vi "Heat Up Macro Prepare Data for Step.vi"(8 "Error In":errorcluster, 10 "Columns Too Search For":string[](array[string])=["System Time", "Draw Elapsed Time (s)", "Elapsed Time (s)", "UE - state (1/0 on off)", "LE - state (1/0 on off)", "Comp - state (1/0 on off)", "Fan  - state (1/0 on off)", "GALLONS", "FLOW(GPM)", "Intellifaucet Valve % Open", "Program Status", "Flow Events (Bit Encoded)"], 11 "HeatUp Raw Data Input":string[][](array[string])) -> (0 "Error Out":errorcluster, 2 "Heat Up Data with Only Selected Columns":string[][](array[string]))   [LabVIEW 2019]
uses:
  <vilib>/Utility/error.llb/DialogType.ctl
panel:
  out "index of element":i32
  out "In-Coming Headers":string[](array[string])
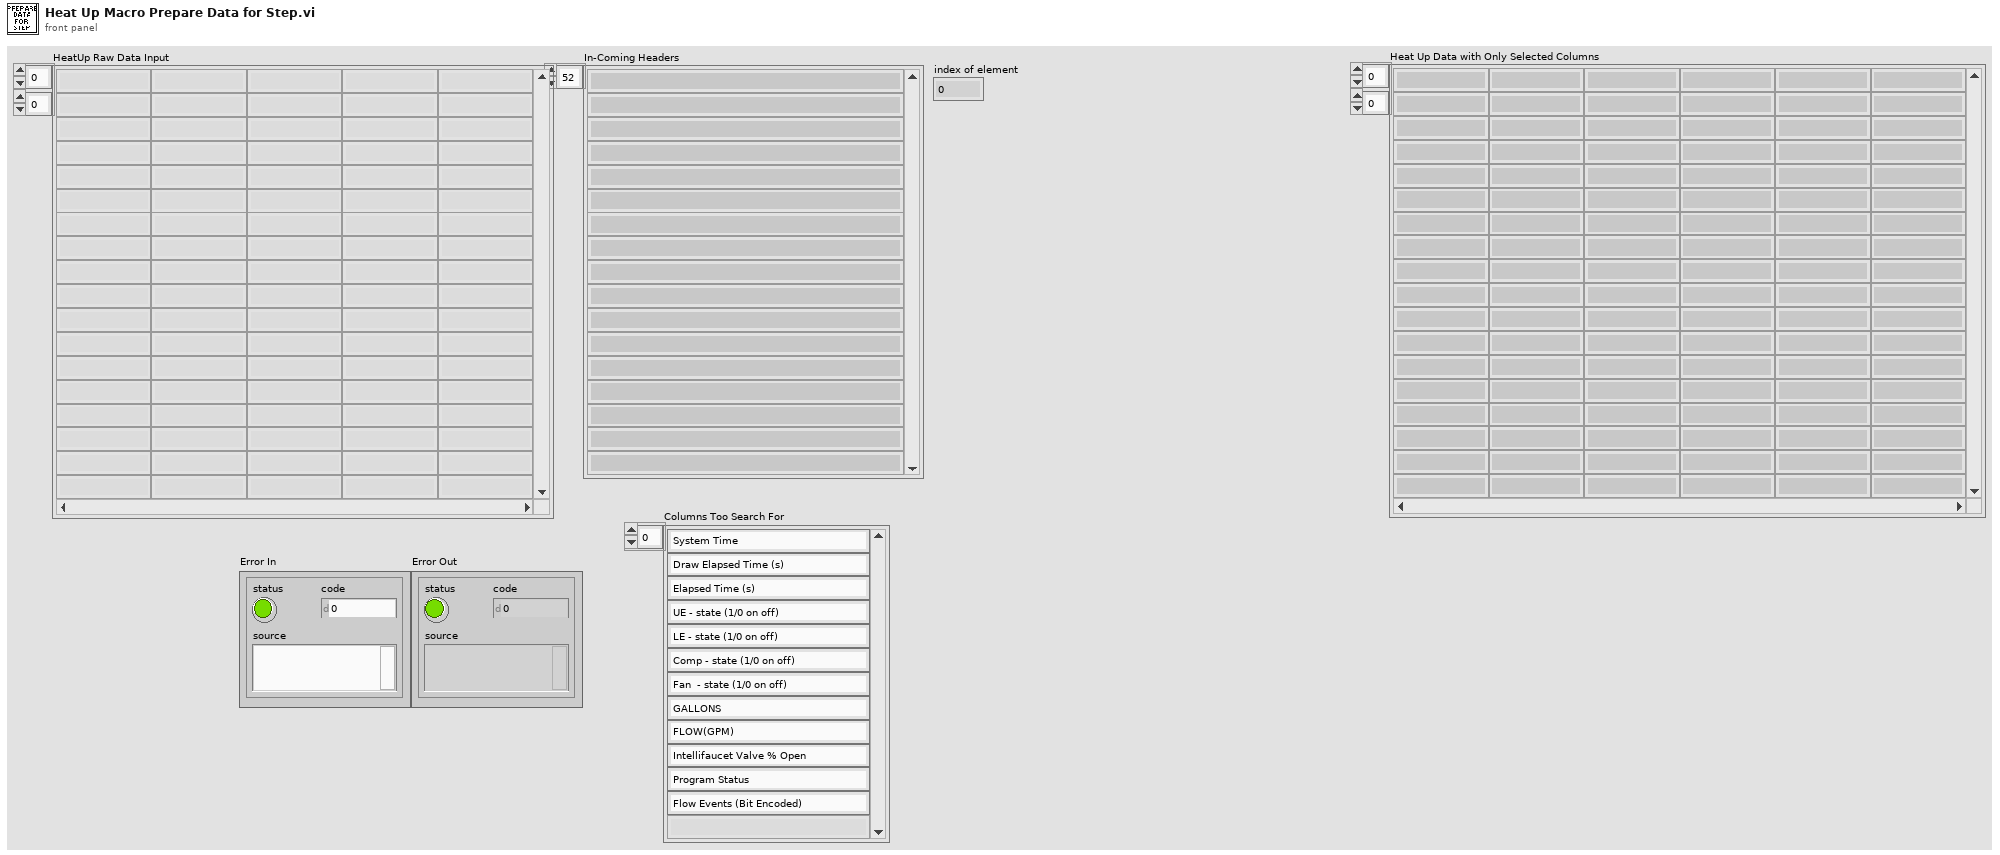
[diagram p1: front panel]
types:
  T1 = typedef "DialogType.ctl" = u16
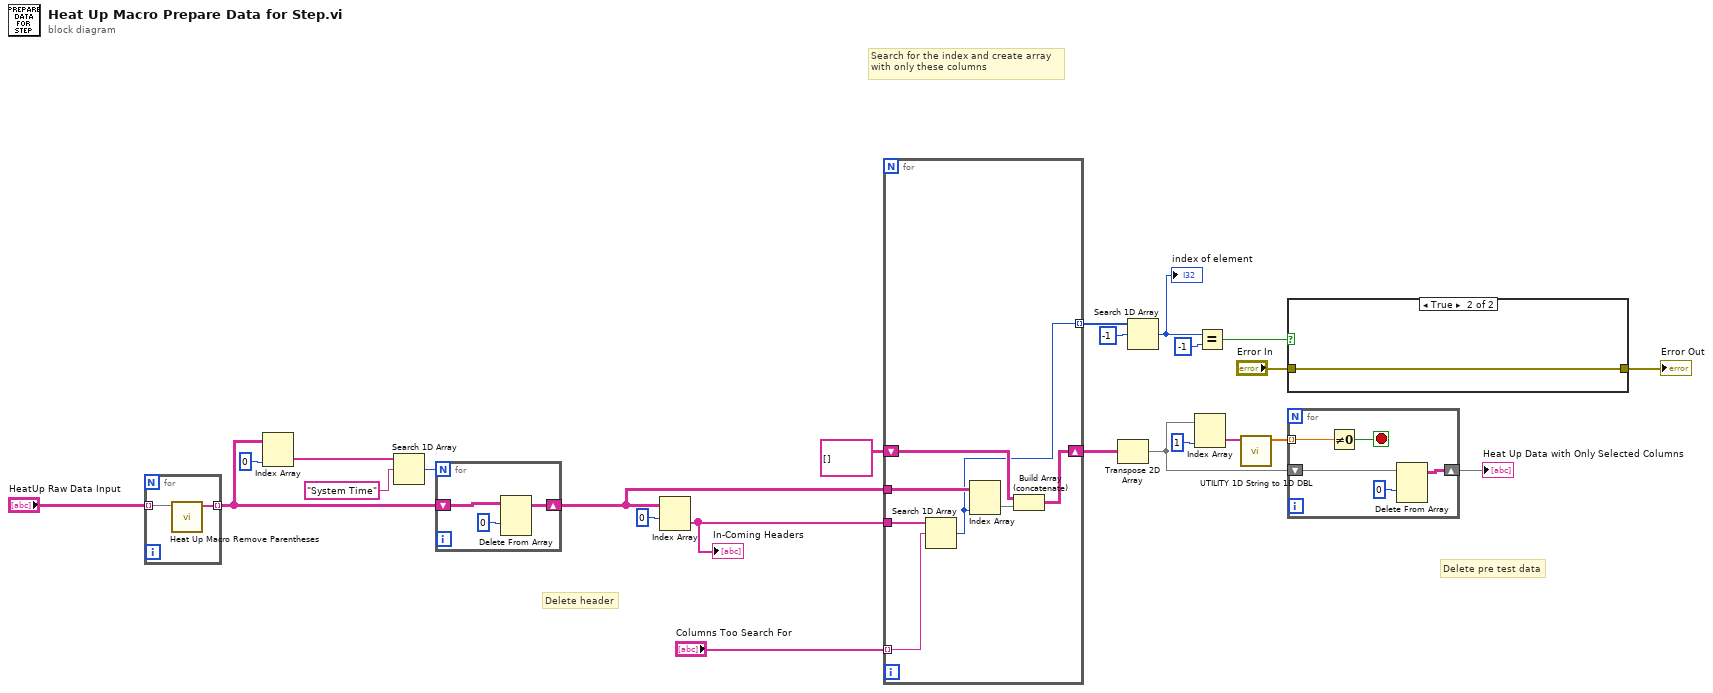
[diagram p0: block diagram]
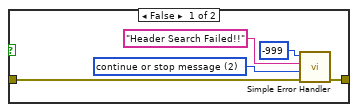
[diagram p2: hidden frame]
diagram:
  # "Delete pre test data"
  # "Delete header"
  # "Search for the index and create array\nwith only these columns"
  n1 = for {
    tunnel: "HeatUp Raw Data Input" -> [w26] mode=indexing
    tunnel: [w25] -> w1 mode=indexing
    n2 = call "Heat Up Macro Remove Parentheses.vi"("Input Array"=w26) -> ("Clean Array"=w25:string[])  [unwired: 10 in]
  }
  n3 = Index Array(array=w1, index (col)=0 ("disabled index (col)")) -> (element=w14:string[])  [unwired: 1 in]
  n4 = Search 1D Array(1D array=w14, element="System Time") -> (index of element=w12:i32)  [unwired: 1 in]
  n5 = for {
    N: w12 -> [_]
    shift-right: [w28] -> w18
    shift-left: w1 -> [w29]
    n6 = Delete From Array(array=w29, index (row)=0) -> (array with subset deleted=w28:string[][])  [unwired: 2 in, 1 out]
  }
  n7 = Index Array(array=w18, index (row)=0) -> (element=w3:string[])  [unwired: 1 in]
  "In-Coming Headers" <- w3
  n8 = for {
    tunnel: w3 -> [w31]
    shift-right: [w35] -> w21
    shift-left: string[][] [] -> [w36]
    tunnel: w18 -> [w34]
    tunnel: "Columns Too Search For" -> [w32] mode=indexing
    tunnel: [w30] -> w10 mode=indexing
    n9 = Search 1D Array(1D array=w31, element=w32) -> (index of element=w30:i32)  [unwired: 1 in]
    n10 = Index Array(array=w34, index (col)=w30) -> (element=w33:string[])  [unwired: 1 in]
    n11 = Build Array (concatenate)(w36, w33) -> (w35:string[][])
  }
  n12 = Transpose 2D Array(2D array=w21) -> (transposed array=w23:string[][])
  n13 = Search 1D Array(1D array=w10, element=-1) -> (index of element=w8:i32)  [unwired: 1 in]
  "index of element" <- w8
  n14 = Index Array(array=w23, index (col)=1 ("disabled index (col)")) -> (element=w20:string[])  [unwired: 1 in]
  n15 = Equal?(x=w8, y=-1) -> (x = y?=w6:bool)
  n16 = call "UTILITY 1D String to 1D DBL.vi"("Save Data"=w20) -> ("DBL"=w22:dbl[])  [unwired: 10 in]
  n17 = case shown="True" w6 {
    tunnel: "Error In" -> [w41 w42]
    tunnel: [w40 w42] -> w5
    frame False {
      w39 = T1 2 items=["no dialog", "OK message", "continue or stop message", "OK message + warnings", "continue/stop + warnings"] ("type of dialog (OK msg:1)")
      n18 = call <vilib>:"Simple Error Handler.vi"("error code (no error:0)"=-999, "error source (\" \")"="Header Search Failed!!" ("error source (\" \")"), "type of dialog (OK msg:1)"=w39, "error in (no error)"=w41) -> ("error out"=w40:errorcluster)  [unwired: 1 in, 4 out]
    }
    frame True {
    }
  }
  "Error Out" <- w5
  n19 = for {
    tunnel: w22 -> [w47] mode=indexing
    shift-right: [w43] -> w24
    shift-left: w23 -> [w45]
    stop <- w46 stop-if-true
    n20 = Not Equal To 0?(x=w47) -> (x != 0?=w46:bool)
    n21 = Delete From Array(array=w45, index (row)=0) -> (array with subset deleted=w43:string[][])  [unwired: 2 in, 1 out]
  }
  "Heat Up Data with Only Selected Columns" <- w24
